vi "WSVCAP SHL FPGA LL Procedure I2C - Read ACK.vi"(0 "Procedure Step":T1, 1 "Wait Ticks Remaining":u32, 7 "I2C Wait Ticks":u32, 9 "Socket Mask":u64 format="%012x", 11 "error in (no error)":errorcluster) -> (3 "Wait Ticks Remaining Out":u32, 4 "Procedure Step Out":T1, 8 "Finished":bool, 10 "ACK Bit Read":u32, 15 "error out":errorcluster)   [LabVIEW 2012]
uses:
  Type Defs/WSVCAP SHL Procedure Step Enum.ctl
  Type Defs/WSVCAP SHL I2C Write Line Enum.ctl
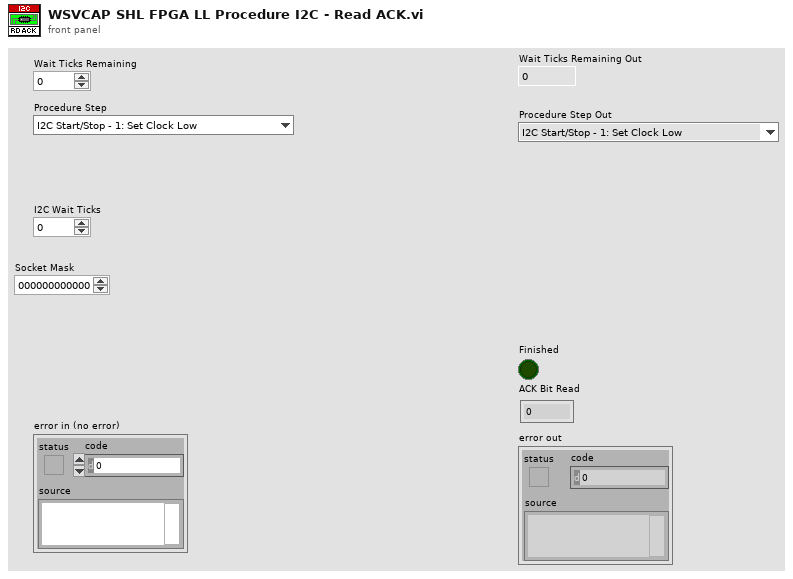
[diagram p1: front panel]
types:
  T1 = typedef "WSVCAP SHL Procedure Step Enum.ctl" = enum16{"I2C Start/Stop - 1: Set Clock Low", "I2C Start/Stop - 2: Wait", "I2C Start/Stop - 3: Set Data I", "I2C Start/Stop - 4: Wait", "I2C Start/Stop - 5: Set Clock High", "I2C Start/Stop - 6: Wait", "I2C Start/Stop - 7: Set Data II", "I2C Start/Stop - 8: Wait", "I2C Start/Stop - 9: Set Clock Low", "I2C Start/Stop - 10: Wait", "I2C Read ACK - 1: Set Clock High", "I2C Read ACK - 2: Wait", "I2C Read ACK - 3: Read ACK Bit", "I2C Read ACK - 4: Wait", "I2C Read ACK - 5: Set Clock Low", "I2C Read ACK - 6: Wait", "I2C Write ACK - 1: Write ACK Bit", "I2C Write ACK - 2: Wait", "I2C Write ACK - 3: Set Clock High", "I2C Write ACK - 4: Wait", "I2C Write ACK - 5: Set Clock Low", "I2C Write ACK - 6: Wait", "I2C Write ACK - 7: Set Data Low", "I2C Send Add - 1: Reset Bits Remaining", "I2C Send Add - 2: Set Data Bit", "I2C Send Add - 3: Wait", "I2C Send Add - 4: Set Clock High", "I2C Send Add - 5: Wait", "I2C Send Add - 6: Set Clock Low", "I2C Send Add - 7: Wait", "I2C Send Add - 8: Check Bits Remaining", "I2C Send Data - 1: Reset Bits Remaining", "I2C Send Data - 2: Load Write Bit from FIFO", "I2C Send Data - 3: Set Data Bit", "I2C Send Data - 4: Wait", "I2C Send Data - 5: Set Clock High", "I2C Send Data - 6: Wait", "I2C Send Data - 7: Set Clock Low", "I2C Send Data - 8: Wait", "I2C Send Data - 9: Check Bits Remaining", "I2C Receive Data - 1: Reset Bits Remaining", "I2C Receive Data - 2: Wait", "I2C Receive Data - 3: Set Clock High", "I2C Receive Data - 4: Wait", "I2C Receive Data - 5: Read Data Bit", "I2C Receive Data - 6: Wait", "I2C Receive Data - 7: Set Clock Low", "I2C Receive Data - 8: Wait", "I2C Receive Data - 9: Check Bits Remaining", "SPI Clear Lines - 1:Clear", "SPI Send/Receive - 1: Load SDA - Clock Low", "SPI Send/Receive - 2: Wait", "SPI Send/Receive - 3: Load DATO - Clock High", "SPI Send/Receive - 4: Wait", "SPI Wait CMD Delay - 1:Wait", "RFFE Send SSC - 1:Set Low", "RFFE Send SSC - 2:Wait", "RFFE Send SSC - 3:Set SDA High", "RFFE Send SSC - 4:Wait", "RFFE Send SSC - 5:Set SDA Low", "RFFE Send SSC - 6:Wait", "RFFE Send Data - 1:Set SCL High", "RFFE Send Data - 2:Wait", "RFFE Send Data - 3:Set SCL Low", "RFFE Send Data - 4:Wait", "RFFE Send Data - 5:Set SCL High (P)", "RFFE Send Data - 6:Wait", "RFFE Send Data - 7:Set SCL Low (P)", "RFFE Send Data - 8:Wait", "RFFE Send Data - 9:Set SCL High (BP)", "RFFE Send Data - 10:Wait", "RFFE Send Data - 11:Set SCL Low (BP)", "RFFE Send Data - 12:Wait", "RFFE Receive Data - 1:Set SCL High", "RFFE Receive Data - 2:Wait", "RFFE Receive Data - 3:Set SCL Low", "RFFE Receive Data - 4:Wait", "RFFE Receive Data - 5:Set SCL High (BP)", "RFFE Receive Data - 6:Wait", "RFFE Receive Data - 7:Set SCL Low (BP)", "RFFE Receive Data - 8:Wait", "RFFE Wait CMD Delay - 1:Wait", "RFFE Clear Lines - 1:Clear"}
  T2 = typedef "WSVCAP SHL I2C Write Line Enum.ctl" = enum16{"I2C SCL", "I2C SDA"}
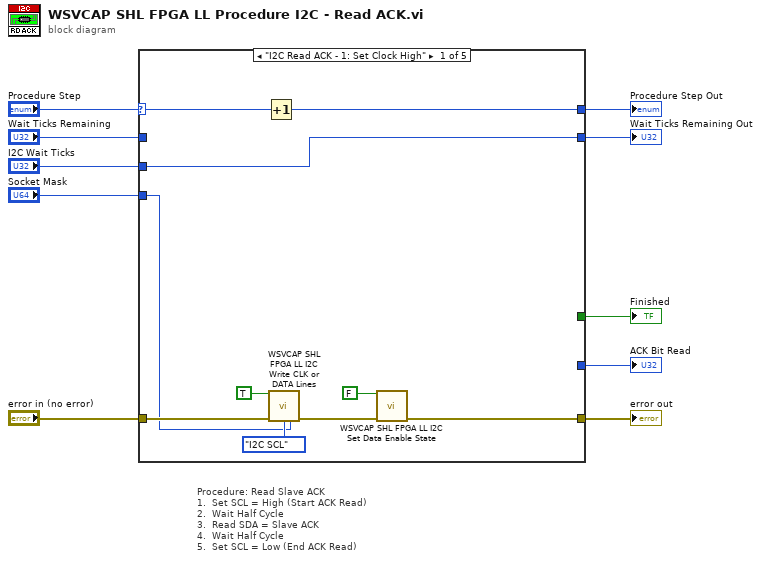
[diagram p0: block diagram]
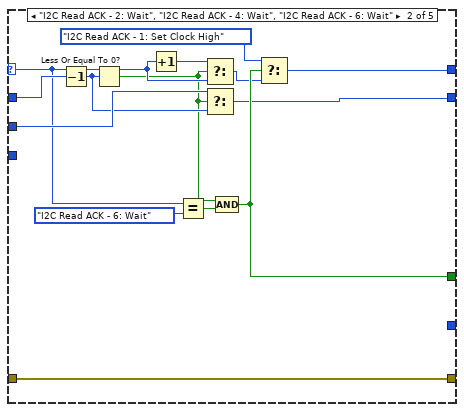
[diagram p2: hidden frame]
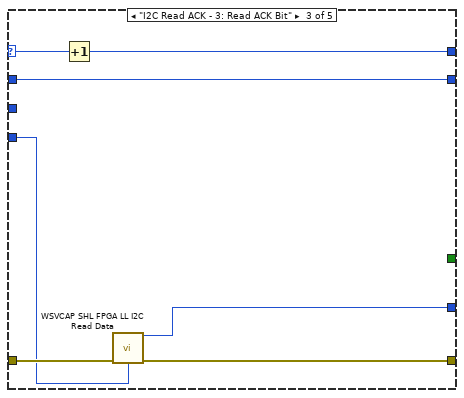
[diagram p3: hidden frame]
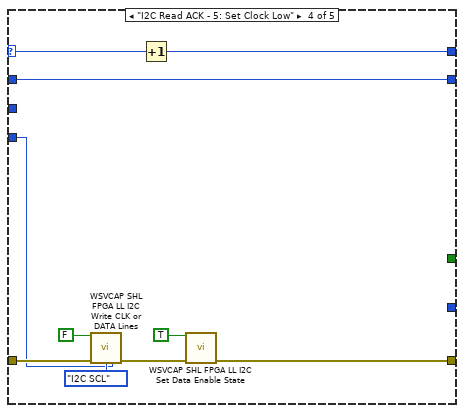
[diagram p4: hidden frame]
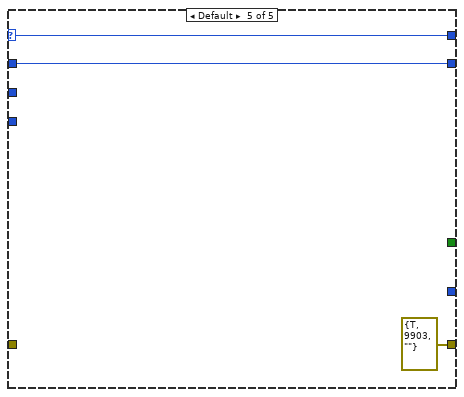
[diagram p5: hidden frame]
diagram:
  # "Procedure: Read Slave ACK\n1.  Set SCL = High (Start ACK Read)\n2.  Wait Half Cycle\n3.  Read SDA = Slave ACK\n4.  Wait Half Cycle\n5.  Set SCL = Low (End ACK Read)"
  n1 = case shown="\"I2C Read ACK - 1: Set Clock High\"" "Procedure Step" {
    selector: "Procedure Step" -> [w17 w29 w39 w45 w53]
    tunnel: [w15 w32 w40 w47 errorcluster {"status"=TRUE, "code"=9903, "source"=""} ("error out")] -> w9
    tunnel: "error in (no error)" -> [w19 w32 w41 w50 _]
    tunnel: "Wait Ticks Remaining" -> [_ w34 w35 w42 w52]
    tunnel: "I2C Wait Ticks" -> [w11 w31 _ _ _]
    tunnel: [_ w26 _ _ _] -> w8
    tunnel: [_ _ w38 _ _] -> w7
    tunnel: "Socket Mask" -> [w13 _ w37 w44 _]
    tunnel: [w11 w22 w35 w42 w52] -> w2
    tunnel: [w12 w21 w36 w43 w53] -> w1
    frame "I2C Read ACK - 1: Set Clock High" {
      n2 = Increment(x=w17) -> (x+1=w12:T1)
      n3 = call "WSVCAP SHL FPGA LL I2C Write CLK or DATA Lines.vi"("Bit In"=TRUE, "error in (no error)"=w19, "Line"=WSVCAP_SHL_I2C_Write_Line_Enum."I2C SCL", "Socket Mask"=w13) -> ("error out"=w16:errorcluster)  [unwired: 11 in]
      n4 = call "WSVCAP SHL FPGA LL I2C Set Data Enable State.vi"("State"=FALSE, "error in (no error)"=w16) -> ("error out"=w15:errorcluster)  [unwired: 13 in]
    }
    frame "I2C Read ACK - 2: Wait", "I2C Read ACK - 4: Wait", "I2C Read ACK - 6: Wait" {
      n5 = Decrement(x=w34) -> (x-1=w30:u32)
      n6 = Less Or Equal To 0?(x=w30) -> (x <= 0?=w28:bool)
      n7 = Increment(x=w29) -> (x+1=w33:T1)
      n8 = Equal?(x=w29, y=WSVCAP_SHL_Procedure_Step_Enum."I2C Read ACK - 6: Wait" ("Procedure Step")) -> (x = y?=w27:bool)
      n9 = Select(t=w33, s=w28, f=w29) -> (s? t:f=w25:T1)
      n10 = Select(t=w31, s=w28, f=w30) -> (s? t:f=w22:u32)
      n11 = Compound Arithmetic op=AND(w28, w27) -> (w26:bool)
      n12 = Select(t=WSVCAP_SHL_Procedure_Step_Enum."I2C Read ACK - 1: Set Clock High" ("Procedure Step"), s=w26, f=w25) -> (s? t:f=w21:T1)
    }
    frame "I2C Read ACK - 3: Read ACK Bit" {
      n13 = Increment(x=w39) -> (x+1=w36:T1)
      n14 = call "WSVCAP SHL FPGA LL I2C Read Data.vi"("error in (no error)"=w41, "Socket Mask"=w37) -> ("Long Word Out (1-Bit for Each Channel)"=w38:u64, "error out"=w40:errorcluster)  [unwired: 12 in]
    }
    frame "I2C Read ACK - 5: Set Clock Low" {
      n15 = call "WSVCAP SHL FPGA LL I2C Write CLK or DATA Lines.vi"("Bit In"=FALSE, "error in (no error)"=w50, "Line"=WSVCAP_SHL_I2C_Write_Line_Enum."I2C SCL", "Socket Mask"=w44) -> ("error out"=w48:errorcluster)  [unwired: 11 in]
      n16 = Increment(x=w45) -> (x+1=w43:T1)
      n17 = call "WSVCAP SHL FPGA LL I2C Set Data Enable State.vi"("State"=TRUE, "error in (no error)"=w48) -> ("error out"=w47:errorcluster)  [unwired: 13 in]
    }
    frame Default {
    }
  }
  "error out" <- w9
  "Finished" <- w8
  "ACK Bit Read" <- w7
  "Wait Ticks Remaining Out" <- w2
  "Procedure Step Out" <- w1
